vi "Remove Dependency.vi"(8 "error in (no error)":errorcluster, 10 "GUID":string, 11 "Attribute.Dependencies in":refnum<class "Attribute.Dependencies.lvclass">) -> (0 "error out":errorcluster, 3 "Attribute.Dependencies out":refnum<class "Attribute.Dependencies.lvclass">)   [LabVIEW 2013, in "Attribute.Dependencies.lvclass"]
uses:
  Attribute.Dependencies.lvclass
  Attribute.Dependencies.lvclass/Attribute.Dependencies.ctl
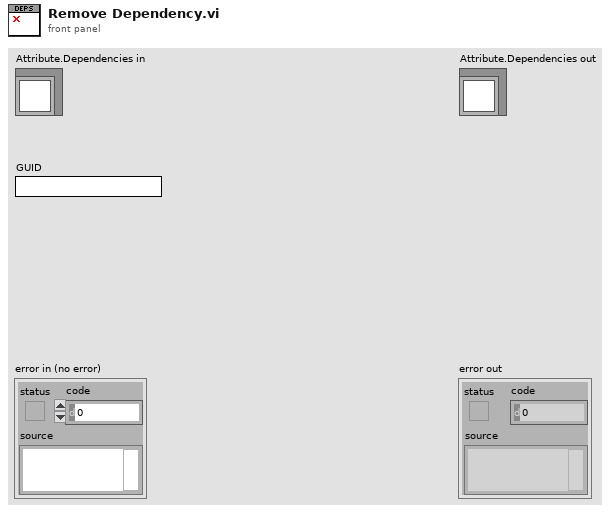
[diagram p1: front panel]
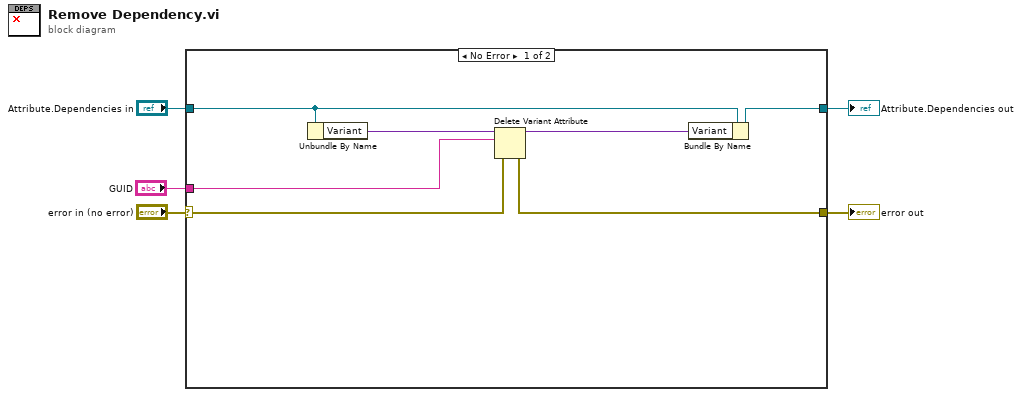
[diagram p0: block diagram]
diagram:
  n1 = case shown="No Error" "error in (no error)" {
    selector: "error in (no error)" -> [w7 w14]
    tunnel: [w6 w14] -> w4
    tunnel: [w12 w13] -> w2
    tunnel: "Attribute.Dependencies in" -> [w11 w13]
    tunnel: "GUID" -> [w10 _]
    frame No Error {
      n2 = Unbundle By Name(w11) -> ("Variant"=w9:variant)
      n3 = Delete Variant Attribute(4:w7, 6:w10, 7:w9) -> (0:w6:errorcluster, 3:w8:variant)  [unwired: 1 out]
      n4 = Bundle By Name(cluster=w11, "Variant"=w8) -> (w12:refnum<class "Attribute.Dependencies.lvclass">)
    }
    frame Error {
    }
  }
  "error out" <- w4
  "Attribute.Dependencies out" <- w2
